vi "cryo_transfer_station.vi"() -> ()   [LabVIEW 2025]
panel:
  in  "100nm":bool
  in  "1um":bool
  in  "10um":bool
  in  "100um":bool
  in  "set z position":dbl min=0.0 max=12.0 step=0.01 format="%_5f"
  in  "set z velocity":dbl=0.16 min=0.0 max=0.16 step=0.01 format="%#_13g"
  in  "set y velocity":dbl=10.0 min=0.0 max=16.0 step=0.01 format="%#_13g"
  in  "set x velocity":dbl=0.16 min=0.0 max=0.16 step=0.01 format="%#_13g"
  in  "set r velocity":dbl=10.0 min=0.0 max=16.0 step=1.0 format="%#_13g"
  out "y position":dbl format="%.3f"
  out "y velocity":dbl format="%.2f"
  in  "set y position":dbl min=0.0 max=12.0 step=0.01 format="%.3f"
  out "x position":dbl format="%.3f"
  out "x velocity":dbl format="%.2f"
  in  "set x position":dbl min=0.0 max=12.0 step=0.01 format="%.3f"
  out "z position":dbl format="%.4f"
  out "z velocity":dbl format="%.2f"
  out "r position":dbl format="%.2f"
  out "r velocity":dbl format="%.2f"
  in  "emergency stop":bool
  in  "set r position":dbl min=-45.0 max=45.0 step=0.1 format="%.2f"
  # "Running this program will home all axes"
  # "Make sure to go slow with z axis, if you set a large value and then try to decrease it the controller sometimes\nhas a delay before registering the new value - this might cause collision between sample and stamp"
  # "max x, y, z positions are 12mm"
  # "max xyz velocity is 0.16, max rotation velocity is 16"
  # "rotation is limited to ±45 degrees"
  # "control rotation with\nf7 and f8"
  # "control x with\ninsert and delete"
  # "control y with\nhome and end"
  # "control z with\npage up and page down"
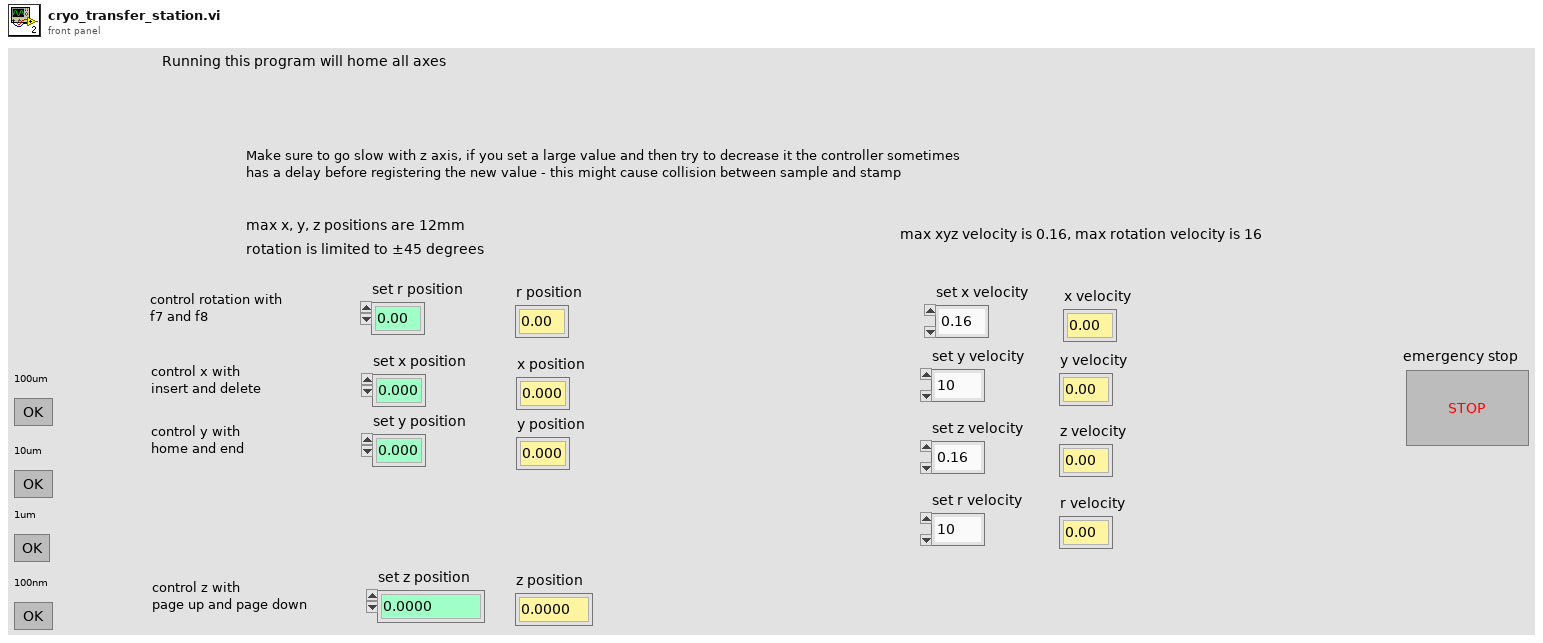
[diagram p1: front panel]
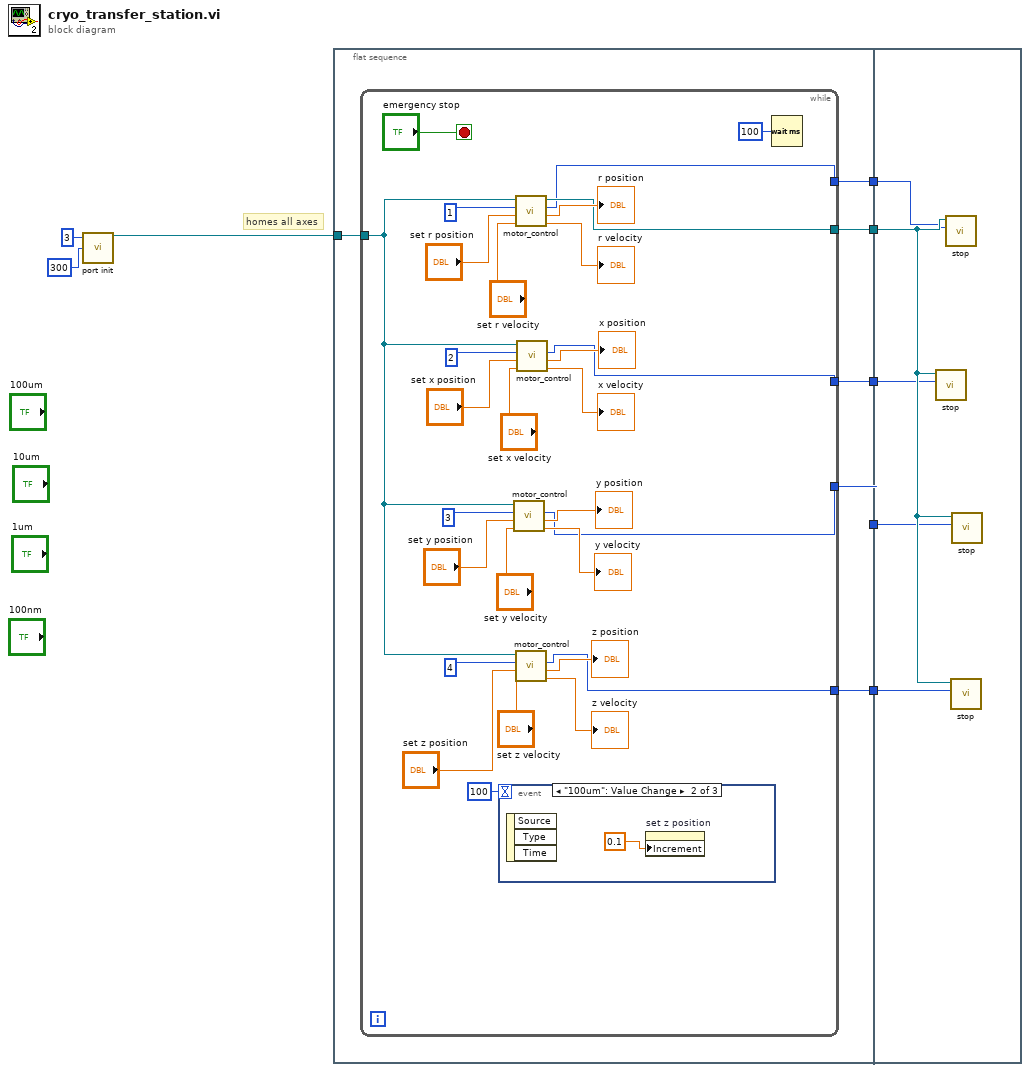
[diagram p0: block diagram]
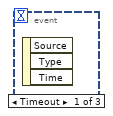
[diagram p2: hidden frame]
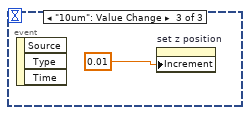
[diagram p3: hidden frame]
diagram:
  # "homes all axes"
  n1 = call <userlib>:"port init.vi"("Timeout (ms)"=u32 300, "SerialPort"=u8 3) -> ("Visa Handle"=w1:refnum<visa-resource-name>)  [unwired: 2 in, 1 out]
  n2 = flat-sequence {
    tunnel: w1 -> [w14]
    tunnel: [w13] -> w6
    tunnel: [w12] -> w5
    tunnel: [w11] -> w4
    tunnel: [w10] -> w3
    tunnel: [w9] -> w2
    tunnel: w6 -> [w50]
    tunnel: w5 -> [w49]
    tunnel: w4 -> [w48]
    tunnel: w3 -> [w47]
    tunnel: w2 -> [w46]
    frame #0 {
      n3 = while {
        tunnel: w14 -> [w24]
        tunnel: [w23] -> w13
        tunnel: [w22] -> w12
        tunnel: [w21] -> w11
        tunnel: [w20] -> w10
        tunnel: [w19] -> w9
        stop <- "emergency stop" stop-if-true
        n4 = event shown="[1] \"100um\": Value Change" {
          selector: _ -> [_ _ _]
          dyn-events: _ -> [_ _ _]
          timeout: 100 -> [_ _ _]
          event Timeout {
            n5 = event-data() -> ()  [unwired: 1 in, 3 out]
          }
          event "100um": Value Change {
            n6 = event-data() -> ()  [unwired: 1 in, 3 out]
            n7 = property on="set z position" class="DigNum (strict)"("Increment"=0.1 ("Data Entry Limits:Increment")) -> ()  [unwired: 2 in, 2 out]
          }
          event "10um": Value Change {
            n8 = event-data() -> ()  [unwired: 1 in, 3 out]
            n9 = property on="set z position" class="DigNum (strict)"("Increment"=0.01 ("Data Entry Limits:Increment")) -> ()  [unwired: 2 in, 2 out]
          }
        }
        n10 = call "motor_control.vi"("set velocity"="set y velocity", "set position"="set y position", "Axis in in"=3, "VISA Refnum in"=w24) -> ("actual velocity"=→"y velocity":dbl, "actual position"=→"y position":dbl, "Axis out"=w20:i32)  [unwired: 4 in, 1 out]
        n11 = call "motor_control.vi"("set velocity"="set r velocity", "set position"="set r position", "Axis in in"=1, "VISA Refnum in"=w24) -> ("actual velocity"=→"r velocity":dbl, "actual position"=→"r position":dbl, "Axis out"=w22:i32, "VISA Handle out"=w23:refnum<visa-resource-name>)  [unwired: 4 in]
        n12 = call "motor_control.vi"("set velocity"="set z velocity", "set position"="set z position", "Axis in in"=4, "VISA Refnum in"=w24) -> ("actual velocity"=→"z velocity":dbl, "actual position"=→"z position":dbl, "Axis out"=w19:i32)  [unwired: 4 in, 1 out]
        n13 = call "motor_control.vi"("set velocity"="set x velocity", "set position"="set x position", "Axis in in"=2, "VISA Refnum in"=w24) -> ("actual velocity"=→"x velocity":dbl, "actual position"=→"x position":dbl, "Axis out"=w21:i32)  [unwired: 4 in, 1 out]
        n14 = Wait (ms)(milliseconds to wait=u32 100) -> ()  [unwired: 1 out]
      }
    }
    frame #1 {
      n15 = call "stop.vi"("Axis in"=w48, "VISA Handle in"=w50) -> ()  [unwired: 4 in, 4 out]
      n16 = call "stop.vi"("Axis in"=w49, "VISA Handle in"=w50) -> ()  [unwired: 4 in, 4 out]
      n17 = call "stop.vi"("Axis in"=w46, "VISA Handle in"=w50) -> ()  [unwired: 4 in, 4 out]
      n18 = call "stop.vi"("Axis in"=w47, "VISA Handle in"=w50) -> ()  [unwired: 4 in, 4 out]
    }
  }
